vi "Tarea03.vi"() -> ()   [LabVIEW 2017]
uses:
  <vilib>/Instr/_visa.llb/VISA Configure Serial Port (Instr).vi
panel:
  out "It's a:":string
  in  "stop":bool
  out "you type":string
  in  "VISA resource name":refnum<visa-resource-name>
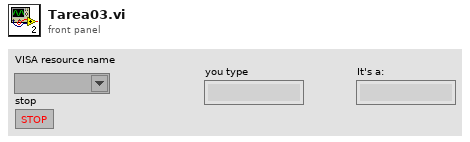
[diagram p1: front panel]
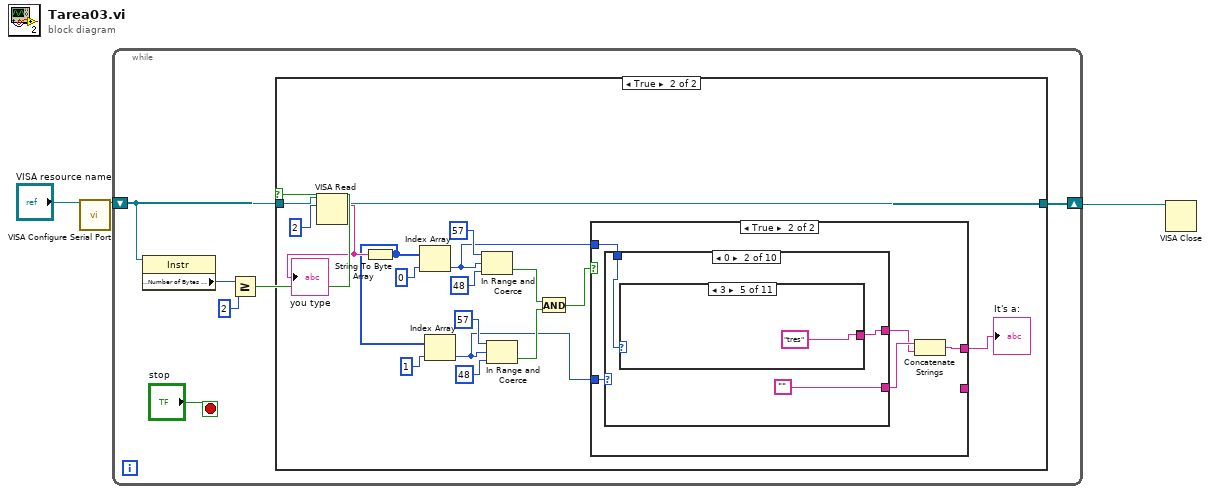
[diagram p0: block diagram]
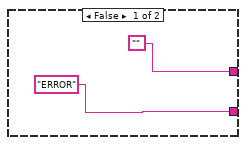
[diagram p3: hidden frame]
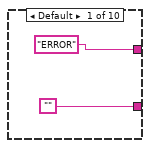
[diagram p4: hidden frame]
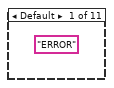
[diagram p5: hidden frame]
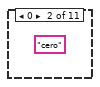
[diagram p6: hidden frame]
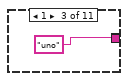
[diagram p7: hidden frame]
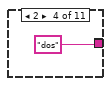
[diagram p8: hidden frame]
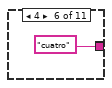
[diagram p9: hidden frame]
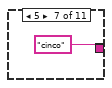
[diagram p10: hidden frame]
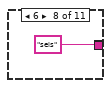
[diagram p11: hidden frame]
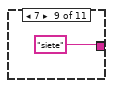
[diagram p12: hidden frame]
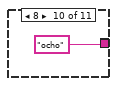
[diagram p13: hidden frame]
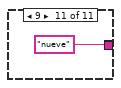
[diagram p14: hidden frame]
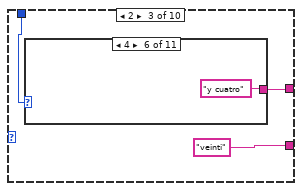
[diagram p15: hidden frame]
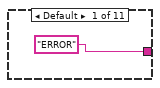
[diagram p16: hidden frame]
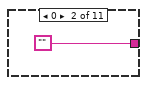
[diagram p17: hidden frame]
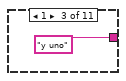
[diagram p18: hidden frame]
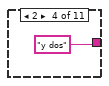
[diagram p19: hidden frame]
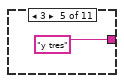
[diagram p20: hidden frame]
diagram:
  n1 = call-poly "VISA Configure Serial Port"("VISA resource name"="VISA resource name") -> ("VISA resource name out"=w2:refnum<visa-resource-name>)  [unwired: 13 in, 1 out]
  n2 = while {
    shift-right: [w9] -> w1
    shift-left: w2 -> [w7]
    stop <- "stop" stop-if-true
    n3 = property class="Instr"(reference=w7) -> ("Serial Settings:Number of Bytes at Serial Port"=w6:u32)  [unwired: 1 in, 2 out]
    n4 = Greater Or Equal?(x=w6, y=u32 2) -> (x >= y?=w4:bool)
    n5 = case shown="True" w4 {
      tunnel: w7 -> [w10 w26]
      tunnel: [w10 w27] -> w9
      frame False {
      }
      frame True {
        n6 = VISA Read(VISA resource name=w26, byte count=u32 2) -> (VISA resource name out=w27:refnum<visa-resource-name>, read buffer=w24:string)  [unwired: 1 in, 2 out]
        "you type" <- w24
        n7 = String To Byte Array(string=w24) -> (unsigned byte array=w17:u8[])
        n8 = Index Array(array=w17, index=0) -> (element=w12:u8)
        n9 = Index Array(array=w17, index=1) -> (element=w13:u8)
        n10 = In Range and Coerce(upper limit=u8 57, x=w12, lower limit=u8 48) -> (In Range?=w16:bool)  [unwired: 1 out]
        n11 = In Range and Coerce(upper limit=u8 57, x=w13, lower limit=u8 48) -> (In Range?=w15:bool)  [unwired: 1 out]
        n12 = And(x=w16, y=w15) -> (x .and. y?=w14:bool)
        n13 = case shown="True" w14 {
          tunnel: ["ERROR" _] -> _
          tunnel: w13 -> [_ w34]
          tunnel: w12 -> [_ w33]
          tunnel: ["" w32] -> w11
          frame False {
          }
          frame True {
            n14 = case shown="0" w34 {
              tunnel: ["" "" "veinti" "treinta y " "cuarenta y " "cincuenta y " "sesenta y " "setenta y " "ochenta y " "noventa y "] -> w31
              tunnel: w33 -> [_ w38 w49 w63 w77 w91 w105 w119 w133 w147]
              tunnel: ["ERROR" w37 w50 w64 w78 w92 w106 w120 w134 w148] -> w30
              frame Default {
              }
              frame 0 {
                n15 = case shown="3" w38 {
                  tunnel: [_ _ "uno" "dos" "tres" _ "cinco" "seis" "siete" "ocho" "nueve"] -> w37
                  tunnel: [_ _ _ _ _ "cuatro" _ _ _ _ _] -> _
                  frame Default {
                    (unwired) "ERROR"
                  }
                  frame 0 {
                    (unwired) "cero"
                  }
                  frame 1 {
                  }
                  frame 2 {
                  }
                  frame 3 {
                  }
                  frame 4 {
                  }
                  frame 5 {
                  }
                  frame 6 {
                  }
                  frame 7 {
                  }
                  frame 8 {
                  }
                  frame 9 {
                  }
                }
              }
              frame 2 {
                n16 = case shown="4" w49 {
                  tunnel: ["ERROR" "" "y uno" "y dos" "y tres" "y cuatro" "y cinco" "y seis" "y siete" "y ocho" "y nueve"] -> w50
                  frame Default {
                  }
                  frame 0 {
                  }
                  frame 1 {
                  }
                  frame 2 {
                  }
                  frame 3 {
                  }
                  frame 4 {
                  }
                  frame 5 {
                  }
                  frame 6 {
                  }
                  frame 7 {
                  }
                  frame 8 {
                  }
                  frame 9 {
                  }
                }
              }
              frame 3 {
                n17 = case shown="4" w63 {
                  tunnel: ["ERROR" "" "y uno" "y dos" "y tres" "y cuatro" "y cinco" "y seis" "y siete" "y ocho" "y nueve"] -> w64
                  frame Default {
                  }
                  frame 0 {
                  }
                  frame 1 {
                  }
                  frame 2 {
                  }
                  frame 3 {
                  }
                  frame 4 {
                  }
                  frame 5 {
                  }
                  frame 6 {
                  }
                  frame 7 {
                  }
                  frame 8 {
                  }
                  frame 9 {
                  }
                }
              }
              frame 4 {
                n18 = case shown="4" w77 {
                  tunnel: ["ERROR" "" "y uno" "y dos" "y tres" "y cuatro" "y cinco" "y seis" "y siete" "y ocho" "y nueve"] -> w78
                  frame Default {
                  }
                  frame 0 {
                  }
                  frame 1 {
                  }
                  frame 2 {
                  }
                  frame 3 {
                  }
                  frame 4 {
                  }
                  frame 5 {
                  }
                  frame 6 {
                  }
                  frame 7 {
                  }
                  frame 8 {
                  }
                  frame 9 {
                  }
                }
              }
              frame 5 {
                n19 = case shown="4" w91 {
                  tunnel: ["ERROR" "" "y uno" "y dos" "y tres" "y cuatro" "y cinco" "y seis" "y siete" "y ocho" "y nueve"] -> w92
                  frame Default {
                  }
                  frame 0 {
                  }
                  frame 1 {
                  }
                  frame 2 {
                  }
                  frame 3 {
                  }
                  frame 4 {
                  }
                  frame 5 {
                  }
                  frame 6 {
                  }
                  frame 7 {
                  }
                  frame 8 {
                  }
                  frame 9 {
                  }
                }
              }
              frame 6 {
                n20 = case shown="4" w105 {
                  tunnel: ["ERROR" "" "y uno" "y dos" "y tres" "y cuatro" "y cinco" "y seis" "y siete" "y ocho" "y nueve"] -> w106
                  frame Default {
                  }
                  frame 0 {
                  }
                  frame 1 {
                  }
                  frame 2 {
                  }
                  frame 3 {
                  }
                  frame 4 {
                  }
                  frame 5 {
                  }
                  frame 6 {
                  }
                  frame 7 {
                  }
                  frame 8 {
                  }
                  frame 9 {
                  }
                }
              }
              frame 7 {
                n21 = case shown="4" w119 {
                  tunnel: ["ERROR" "" "y uno" "y dos" "y tres" "y cuatro" "y cinco" "y seis" "y siete" "y ocho" "y nueve"] -> w120
                  frame Default {
                  }
                  frame 0 {
                  }
                  frame 1 {
                  }
                  frame 2 {
                  }
                  frame 3 {
                  }
                  frame 4 {
                  }
                  frame 5 {
                  }
                  frame 6 {
                  }
                  frame 7 {
                  }
                  frame 8 {
                  }
                  frame 9 {
                  }
                }
              }
              frame 8 {
                n22 = case shown="4" w133 {
                  tunnel: ["ERROR" "" "y uno" "y dos" "y tres" "y cuatro" "y cinco" "y seis" "y siete" "y ocho" "y nueve"] -> w134
                  frame Default {
                  }
                  frame 0 {
                  }
                  frame 1 {
                  }
                  frame 2 {
                  }
                  frame 3 {
                  }
                  frame 4 {
                  }
                  frame 5 {
                  }
                  frame 6 {
                  }
                  frame 7 {
                  }
                  frame 8 {
                  }
                  frame 9 {
                  }
                }
              }
              frame 9 {
                n23 = case shown="4" w147 {
                  tunnel: ["ERROR" "" "y uno" "y dos" "y tres" "y cuatro" "y cinco" "y seis" "y siete" "y ocho" "y nueve"] -> w148
                  frame Default {
                  }
                  frame 0 {
                  }
                  frame 1 {
                  }
                  frame 2 {
                  }
                  frame 3 {
                  }
                  frame 4 {
                  }
                  frame 5 {
                  }
                  frame 6 {
                  }
                  frame 7 {
                  }
                  frame 8 {
                  }
                  frame 9 {
                  }
                }
              }
            }
            n24 = Concatenate Strings(w31, w30) -> (w32:string)
          }
        }
        "It's a:" <- w11
      }
    }
  }
  n25 = VISA Close(VISA resource name=w1) -> ()  [unwired: 1 in, 1 out]
